vi "Read Main CD Properties.vi"(8 "error in (no error)":errorcluster, 11 "CustomDevice in":refnum<class "CustomDevice.lvclass">) -> (0 "error out":errorcluster, 2 "Main CD Properties":T1, 3 "CustomDevice out":refnum<class "CustomDevice.lvclass">)   [LabVIEW 2015, in "CustomDevice.lvclass"]
uses:
  CustomDevice.lvclass
  XML Controls/Main Custom Device Properties.ctl
  CustomDevice.lvclass/CustomDevice.ctl
  VeriStand XML Parser.lvlib
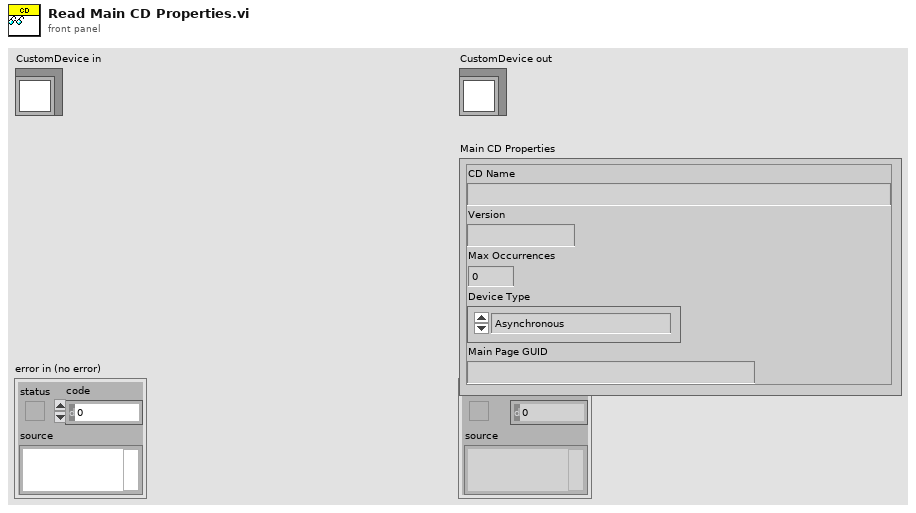
[diagram p1: front panel]
types:
  T1 = typedef "VeriStand XML Parser.lvlib/Main Custom Device Properties.ctl" = cluster{"CD Name":string, "Version":string, "Max Occurrences":i32, "Device Type":enum16{"Asynchronous", "Inline HW Interface", "Inline Model Interface", "Inline Timing and Sync", "Asynchronous Timing and Sync"}, "Main Page GUID":string}
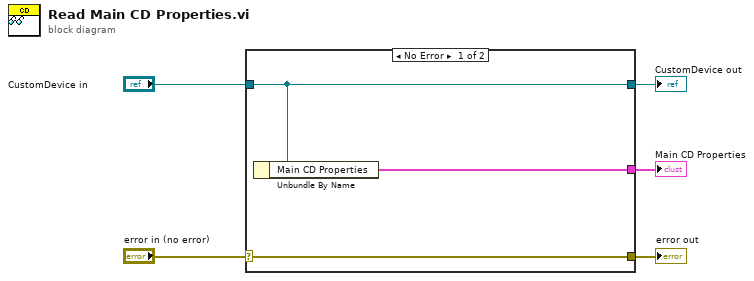
[diagram p0: block diagram]
diagram:
  n1 = case shown="No Error" "error in (no error)" {
    selector: "error in (no error)" -> [w8 w9]
    tunnel: [w8 w9] -> w4
    tunnel: [w7 w10] -> w2
    tunnel: "CustomDevice in" -> [w7 w10]
    tunnel: [w6 _] -> w1
    frame No Error {
      n2 = Unbundle By Name(w7) -> ("Main CD Properties"=w6:T1)
    }
    frame Error {
    }
  }
  "error out" <- w4
  "CustomDevice out" <- w2
  "Main CD Properties" <- w1
